vi "Consumer.vi"(8 "error in (no error)":errorcluster, 9 "Data":variant, 10 "Case ID":string, 11 "uService Template in":refnum<class "TCP Writer.lvclass">) -> (0 "error out":errorcluster, 3 "uService Template out":refnum<class "TCP Writer.lvclass">)   [LabVIEW 2026, in "TALOS.lvlib" / "TCP Writer.lvlib" / "TCP Writer.lvclass"]
uses:
  TCP Writer.lvclass
  C:/LabVIEW Code/TALOS/talos/Father of all uServices/Father of all uServices/Father of all uServices.lvclass
  TCP Writer Consumer Case Selector.ctl
  TCP Writer.lvclass/TCP Writer.ctl
  Father of all uServices/Father of all uServices Messages/Consumer Msg/Consumer Msg.lvclass/Consumer Msg.ctl
  Ancestor/Ancestor/Ancestor.lvclass/Ancestor.ctl
  Father of all uServices/Father of all uServices/Father of all uServices.lvclass/Father of all uServices.ctl
  Ancestor/Ancestor/Infinite Message Selector.ctl
  Support VIs/Generate Error.vi
  FGV/Error Memory/Get Error Description.vi
  Ancestor/Ancestor/Read ID.vi
  Support VIs/Get Class Name.vi
  FGV/Error Memory/Error Memory Core.vi
  <vilib>/AdvancedString/Delimited String to 1D String Array.vi
  <vilib>/AdvancedString/Delimited String to 1D String Array (string).vi
  Support VIs/Circus Root Path.vi
  FGV/Error Memory/Error Crt Lvl checker.vi
  FGV/Error Memory/Error Memory Core.vi/40c8088d-b597-4017-91af-faa98e00292e.vi
  FGV/Error Memory/Error Memory Core.vi/d4a3ab98-063c-4e44-b43d-fbdcfe6c2be2.vi
  Father of all uServices/Father of all uServices/Father of all uServices.lvclass
  C:/LabVIEW Code/TALOS/builds/Actor Framework PPL/Actor Framework.lvlibp/1abvi3w/vi.lib/ActorFramework/Actor/Actor.lvclass
  builds/Actor Framework PPL/Actor Framework.lvlibp/1abvi3w/vi.lib/ActorFramework/Actor/Read Self Enqueuer.vi
  <userlib>/_OpenG.lib/lvdata/lvdata.llb/Get Strings from Enum__ogtk.vi
  builds/Actor Framework PPL/Actor Framework.lvlibp/1abvi3w/vi.lib/ActorFramework/Message Enqueuer/Enqueue.vi
  Support VIs/Global Memory.vi
  <vilib>/Utility/LVClass/Get LV Class Name.vi
  Support VIs/Is in Packed Library.vi
  Support VIs/TALOS Root path.vi
  Support VIs/Read CSV worksheet.vi
  Support VIs/Global Constants.vi
  <vilib>/Utility/error.llb/General Error Handler.vi
  Support VIs/Error Log.vi
  Father of all uServices/Father of all uServices Messages/Consumer Msg/Consumer Msg.lvclass
  Ancestor/Ancestor/Ancestor.lvclass
  <vilib>/Comparison/Equal/Equal Functor/Equal Functor.lvclass
  TALOS.lvlib
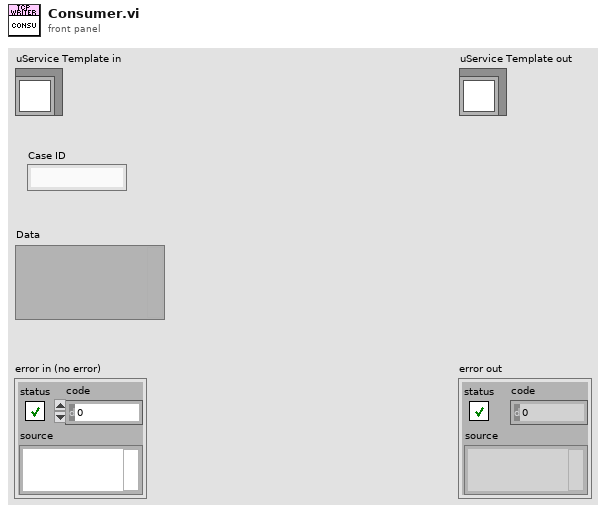
[diagram p1: front panel]
types:
  T1 = typedef "TALOS.lvlib/TCP Writer.lvlib/TCP Writer.lvclass/TCP Writer Consumer Case Selector.ctl" = enum16{"Send message", "Idle", "Check Connection", "Open connection", "Set Client ID"}
  T2 = typedef "TALOS.lvlib/Ancestor.lvlib/Ancestor.lvclass/Infinite Message Selector.ctl" = enum16{"Start", "Stop", "Check", "Flush (Stop all)", "Init"}
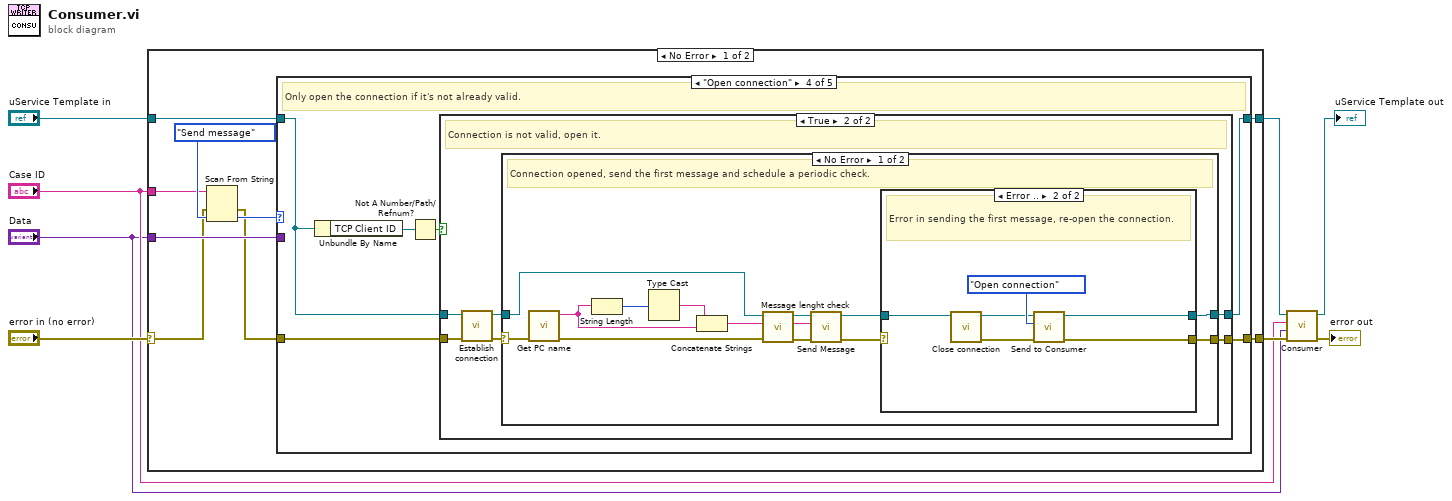
[diagram p0: block diagram]
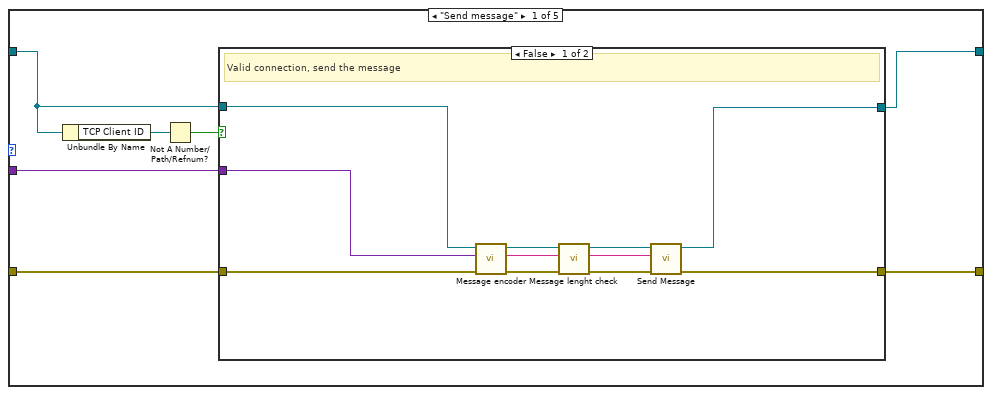
[diagram p2: hidden frame]
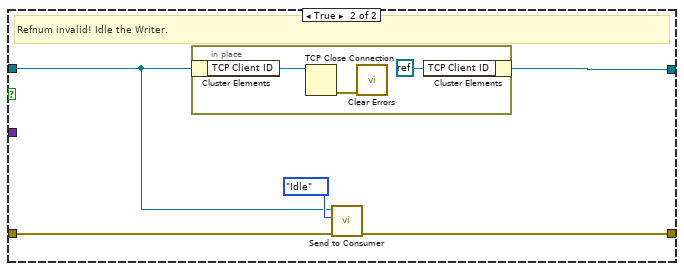
[diagram p3: hidden frame]
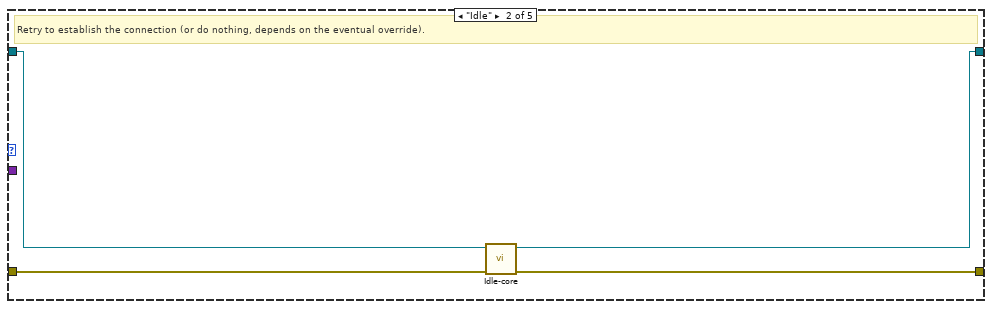
[diagram p4: hidden frame]
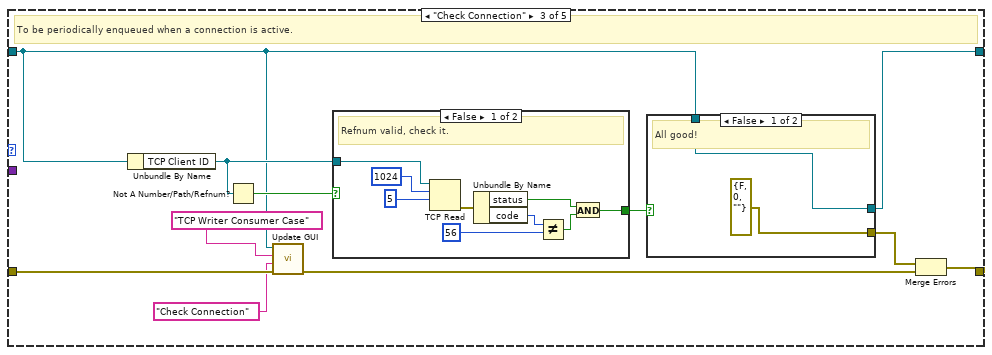
[diagram p5: hidden frame]
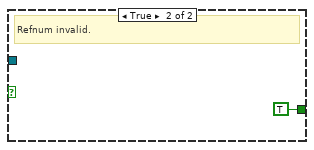
[diagram p6: hidden frame]
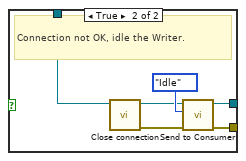
[diagram p7: hidden frame]
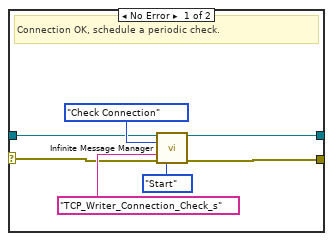
[diagram p9: hidden frame]
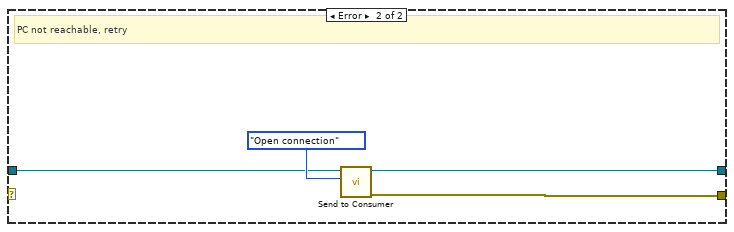
[diagram p10: hidden frame]
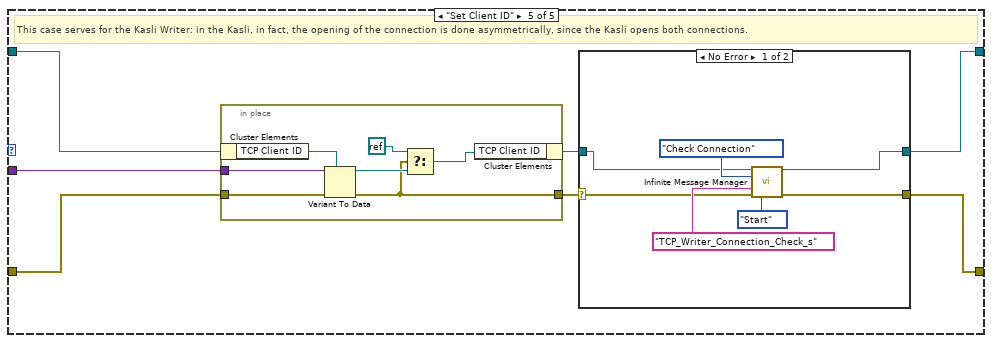
[diagram p11: hidden frame]
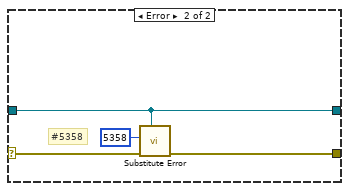
[diagram p12: hidden frame]
diagram:
  n1 = case shown="No Error" "error in (no error)" {
    selector: "error in (no error)" -> [w13 w146]
    tunnel: "uService Template in" -> [w12 w147]
    tunnel: [w15 w147] -> w4
    tunnel: [w16 w146] -> w3
    tunnel: "Case ID" -> [w10 _]
    tunnel: "Data" -> [w17 _]
    frame No Error {
      n2 = Scan From String(input string=w10, error in=w13, default 1=TCP_Writer_Consumer_Case_Selector."Send message") -> (error out=w9:errorcluster, output 1=w11:T1)  [unwired: 2 in, 2 out]
      n3 = case shown="\"Open connection\"" w11 {
        tunnel: w17 -> [w22 _ _ _ w123]
        tunnel: w9 -> [w21 w44 w54 w82 w122]
        tunnel: w12 -> [w23 w47 w48 w79 w125]
        tunnel: [w24 w46 w53 w80 w121] -> w16
        tunnel: [w18 w45 w49 w81 w124] -> w15
        frame "Send message" {
          n4 = Unbundle By Name(w23) -> ("TCP Client ID"=w20:refnum<k5>)
          n5 = Not A Number/Path/Refnum?(number/path/refnum=w20) -> (NaN/Path/Refnum?=w19:bool)
          n6 = case shown="False" w19 {
            tunnel: [w35 w38] -> w24
            tunnel: w23 -> [w34 w37]
            tunnel: w22 -> [w33 _]
            tunnel: w21 -> [w32 w39]
            tunnel: [w28 w36] -> w18
            frame False {
              # "Valid connection, send the message"
              n7 = call-dynamic "Message encoder.vi"("error in (no error)"=w32, "Data"=w33, "TCP Writer in"=w34) -> ("error out"=w31:errorcluster, "Message encoded"=w29:string, "TCP Writer out"=w30:refnum<class "TCP Writer.lvclass">)  [unwired: 6 in]
              n8 = call-dynamic "Message lenght check.vi"("error in (no error)"=w31, "String in"=w29, "TCP Writer in"=w30) -> ("error out"=w27:errorcluster, "String out"=w26:string, "TCP Writer out"=w25:refnum<class "TCP Writer.lvclass">)  [unwired: 6 in]
              n9 = call-dynamic "Send Message.vi"("error in (no error)"=w27, "String in"=w26, "TCP Writer in"=w25) -> ("error out"=w35:errorcluster, "TCP Writer out"=w28:refnum<class "TCP Writer.lvclass">)  [unwired: 7 in]
            }
            frame True {
              # "Refnum invalid! Idle the Writer."
              n10 = in-place {
                n11 = in-place-cluster #1(w37) -> ("TCP Client ID"=w43:refnum<k5>)
                n12 = TCP Close Connection(connection ID=w43) -> (error out=w42:errorcluster)  [unwired: 2 in, 1 out]
                n13 = call <vilib>:"Clear Errors.vi"("error in (no error)"=w42) -> ()  [unwired: 5 in, 2 out]
                n14 = in-place-cluster #1("TCP Client ID"=refnum<k0> refnum) -> (w36:refnum<class "TCP Writer.lvclass">)
              }
              n15 = call "Send to Consumer.vi"("error in (no error)"=w39, "Case ID"=TCP_Writer_Consumer_Case_Selector."Idle" ("TCP Listener Consumer Case Selector"), "uService Template in"=w37) -> ("error out"=w38:errorcluster)  [unwired: 7 in, 1 out]
            }
          }
        }
        frame "Idle" {
          # "Retry to establish the connection (or do nothing, depends on the eventual override)."
          n16 = call-dynamic "Idle-core.vi"("error in (no error)"=w44, "TCP Writer in"=w47) -> ("error out"=w46:errorcluster, "TCP Writer out"=w45:refnum<class "TCP Writer.lvclass">)  [unwired: 8 in]
        }
        frame "Check Connection" {
          # "To be periodically enqueued when a connection is active."
          n17 = Unbundle By Name(w48) -> ("TCP Client ID"=w51:refnum<k5>)
          n18 = Not A Number/Path/Refnum?(number/path/refnum=w51) -> (NaN/Path/Refnum?=w52:bool)
          n19 = call "Update GUI.vi"("error in (no error)"=w54, "Data"="Check Connection", "GUI Item Name"="TCP Writer Consumer Case", "uService Template in"=w48) -> ("error out"=w57:errorcluster)  [unwired: 6 in, 1 out]
          n20 = case shown="False" w52 {
            tunnel: w51 -> [w67 _]
            tunnel: [w62 TRUE] -> w58
            frame False {
              # "Refnum valid, check it."
              n21 = TCP Read(connection ID=w67, bytes to read=1024, 9:5 ("timeout ms (25000)")) -> (error out=w66:errorcluster)  [unwired: 2 in, 2 out]
              n22 = Unbundle By Name(w66) -> ("status"=w63:bool, "code"=w65:i32)
              n23 = Not Equal?(x=w65, y=56) -> (x != y?=w64:bool)
              n24 = And(x=w63, y=w64) -> (x .and. y?=w62:bool)
            }
            frame True {
              # "Refnum invalid."
            }
          }
          n25 = case shown="False" w58 {
            tunnel: w48 -> [w69 w74]
            tunnel: [errorcluster {"status"=FALSE, "code"=0, "source"=""} ("error out") w75] -> w56
            tunnel: [w69 w71] -> w49
            frame False {
              # "All good!"
            }
            frame True {
              # "Connection not OK, idle the Writer."
              n26 = call-dynamic "Close connection.vi"("TCP Writer in"=w74) -> ("error out"=w72:errorcluster, "TCP Writer out"=w73:refnum<class "TCP Writer.lvclass">)  [unwired: 9 in]
              n27 = call "Send to Consumer.vi"("error in (no error)"=w72, "Case ID"=TCP_Writer_Consumer_Case_Selector."Idle" ("TCP Listener Consumer Case Selector"), "uService Template in"=w73) -> ("error out"=w75:errorcluster, "uService Template out"=w71:refnum<class "TCP Writer.lvclass">)  [unwired: 7 in]
            }
          }
          n28 = Merge Errors(w56, w57) -> (w53:errorcluster)
        }
        frame "Open connection" {
          # "Only open the connection if it's not already valid."
          n29 = Unbundle By Name(w79) -> ("TCP Client ID"=w78:refnum<k5>)
          n30 = Not A Number/Path/Refnum?(number/path/refnum=w78) -> (NaN/Path/Refnum?=w77:bool)
          n31 = case shown="True" w77 {
            tunnel: w82 -> [w83 w88]
            tunnel: w79 -> [w84 w86]
            tunnel: [w84 w90] -> w81
            tunnel: [w83 w89] -> w80
            frame False {
              # "Connection is already valid, do not open it!"
            }
            frame True {
              # "Connection is not valid, open it."
              n32 = call-dynamic "Establish connection.vi"("error in (no error)"=w88, "TCP Writer in"=w86) -> ("error out"=w85:errorcluster, "output cluster"=w87:refnum<class "TCP Writer.lvclass">)  [unwired: 8 in]
              n33 = case shown="No Error" w85 {
                selector: w85 -> [w97 _]
                tunnel: w87 -> [w91 w118]
                tunnel: [w104 w117] -> w90
                tunnel: [w103 w119] -> w89
                frame No Error {
                  # "Connection opened, send the first message and schedule a periodic check."
                  n34 = call "Get PC name.vi"("error in (no error)"=w97) -> ("error out"=w92:errorcluster, "Hostname"=w94:string)  [unwired: 9 in]
                  n35 = String Length(string=w94) -> (length=w96:i32)
                  n36 = Type Cast(x=w96) -> (*(type *) &x=w95:string)  [unwired: 1 in]
                  n37 = Concatenate Strings(w95, w94) -> (w93:string)
                  n38 = call-dynamic "Message lenght check.vi"("error in (no error)"=w92, "String in"=w93, "TCP Writer in"=w91) -> ("error out"=w102:errorcluster, "String out"=w101:string, "TCP Writer out"=w100:refnum<class "TCP Writer.lvclass">)  [unwired: 6 in]
                  n39 = call-dynamic "Send Message.vi"("error in (no error)"=w102, "String in"=w101, "TCP Writer in"=w100) -> ("error out"=w98:errorcluster, "TCP Writer out"=w99:refnum<class "TCP Writer.lvclass">)  [unwired: 7 in]
                  n40 = case shown="Error .." w98 {
                    selector: w98 -> [w107 _]
                    tunnel: w99 -> [w105 w114]
                    tunnel: [w109 w113] -> w104
                    tunnel: [w108 w115] -> w103
                    frame No Error {
                      # "Connection OK, schedule a periodic check."
                      n41 = call-dynamic "Infinite Message Manager.vi"("Father of all uServices in"=w105, "Consumer Case Selector"=TCP_Writer_Consumer_Case_Selector."Check Connection", "Tau parameter"="TCP_Writer_Connection_Check_s", "error in (no error)"=w107, "Infinite Message Selector"=Infinite_Message_Selector."Start") -> ("Father of all uServices out"=w109:refnum<class "TCP Writer.lvclass">, "error out"=w108:errorcluster)  [unwired: 8 in, 1 out]
                    }
                    frame Error {
                      # "Error in sending the first message, re-open the connection."
                      n42 = call-dynamic "Close connection.vi"("TCP Writer in"=w114) -> ("error out"=w112:errorcluster, "TCP Writer out"=w113:refnum<class "TCP Writer.lvclass">)  [unwired: 9 in]
                      n43 = call "Send to Consumer.vi"("error in (no error)"=w112, "Case ID"=TCP_Writer_Consumer_Case_Selector."Open connection" ("TCP Listener Consumer Case Selector"), "uService Template in"=w113) -> ("error out"=w115:errorcluster)  [unwired: 7 in, 1 out]
                    }
                  }
                }
                frame Error {
                  # "PC not reachable, retry"
                  n44 = call "Send to Consumer.vi"("Case ID"=TCP_Writer_Consumer_Case_Selector."Open connection" ("TCP Listener Consumer Case Selector"), "uService Template in"=w118) -> ("error out"=w119:errorcluster, "uService Template out"=w117:refnum<class "TCP Writer.lvclass">)  [unwired: 8 in]
                }
              }
            }
          }
        }
        frame "Set Client ID" {
          # "This case serves for the Kasli Writer: in the Kasli, in fact, the opening of the connection is done asymmetrically, since the Kasli opens both connections."
          n45 = in-place "In Place Element Structure" {
            in-place-border: w123 -> [w145]
            in-place-border: w122 -> [w144]
            in-place-border: [w140] -> w127
            n46 = in-place-cluster #2(w125) -> ("TCP Client ID"=w141:refnum<k5>)
            n47 = Variant To Data(error in=w144, type=w141, Variant=w145) -> (data=w143:refnum<k5>, error out=w140:errorcluster)
            n48 = Select(t=refnum<k0> refnum, s=w140, f=w143) -> (s? t:f=w142:refnum<k5>)
            n49 = in-place-cluster #2("TCP Client ID"=w142) -> (w126:refnum<class "TCP Writer.lvclass">)
          }
          n50 = case shown="No Error" w127 {
            selector: w127 -> [w131 w137]
            tunnel: [w130 w136] -> w121
            tunnel: w126 -> [w129 w135]
            tunnel: [w128 w135] -> w124
            frame No Error {
              n51 = call-dynamic "Infinite Message Manager.vi"("Father of all uServices in"=w129, "Consumer Case Selector"=TCP_Writer_Consumer_Case_Selector."Check Connection", "Tau parameter"="TCP_Writer_Connection_Check_s", "error in (no error)"=w131, "Infinite Message Selector"=Infinite_Message_Selector."Start") -> ("Father of all uServices out"=w128:refnum<class "TCP Writer.lvclass">, "error out"=w130:errorcluster)  [unwired: 8 in, 1 out]
            }
            frame Error {
              # "#5358"
              n52 = call "Substitute Error.vi"("LabVIEW Object"=w135, "error in (no error)"=w137, "Error Code"=5358) -> ("error out"=w136:errorcluster)  [unwired: 8 in]
            }
          }
        }
      }
    }
    frame Error {
    }
  }
  n53 = call-parent "Consumer.vi"("error in (no error)"=w3, "Data"="Data", "Case ID"="Case ID", "uService Template in"=w4) -> ("error out"=→"error out":errorcluster, "uService Template out"=→"uService Template out":refnum<class "TCP Writer.lvclass">)  [unwired: 6 in]
